vi "dataReferances.vi"(8 "error in (no error)":errorcluster) -> (0 "error out":errorcluster, 3 "?":T1)   [LabVIEW 2024]
uses:
  controls/dataRefs.ctl
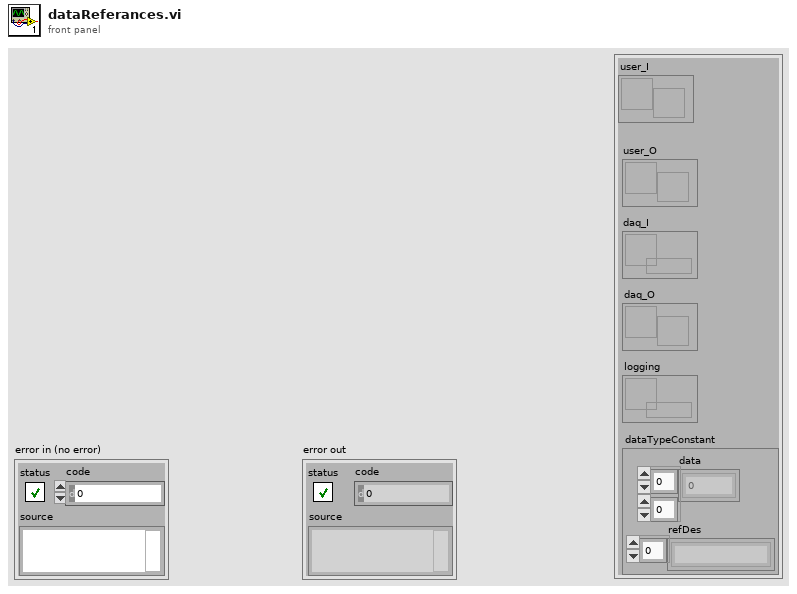
[diagram p1: front panel]
types:
  T1 = typedef "dataRefs.ctl" = cluster{"dataTypeConstant":cluster{"data":dbl[][], "refDes":string[]}, "user_I":refnum<notifier>, "user_O":refnum<notifier>, "daq_O":refnum<notifier>, "logging":refnum<queue>, "daq_I":refnum<queue>}
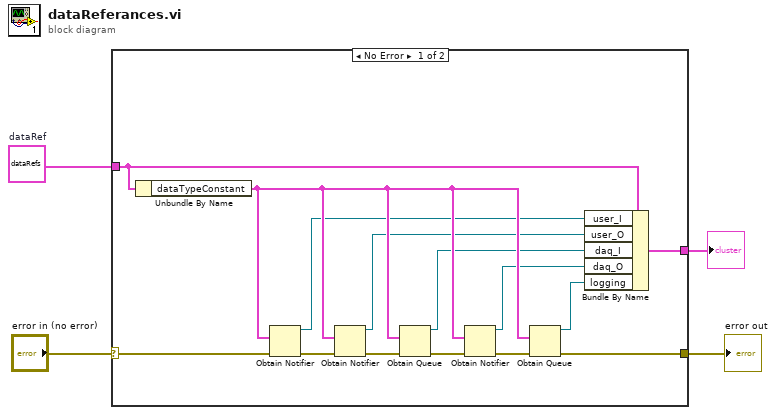
[diagram p0: block diagram]
diagram:
  w1 = T1 {"dataTypeConstant"={"data"=[], "refDes"=[]}, "user_I"=refnum, "user_O"=refnum, "daq_O"=refnum, "logging"=refnum, "daq_I"=refnum}  # dataRef
  n1 = case shown="No Error" "error in (no error)" {
    selector: "error in (no error)" -> [w18 w20]
    tunnel: [w17 w20] -> w3
    tunnel: [w12 w19] -> w2
    tunnel: w1 -> [w11 w19]
    frame No Error {
      n2 = Unbundle By Name(w11) -> ("dataTypeConstant"=w10:cluster{"data":dbl[][], "refDes":string[]})
      n3 = Obtain Notifier(notification data type=w10, error in (no error)=w18) -> (notifier out=w9:refnum<notifier>, error out=w16:errorcluster)  [unwired: 2 in, 1 out]
      n4 = Obtain Notifier(notification data type=w10, error in (no error)=w16) -> (notifier out=w8:refnum<notifier>, error out=w15:errorcluster)  [unwired: 2 in, 1 out]
      n5 = Obtain Queue(element data type=w10, error in (no error)=w15) -> (queue out=w6:refnum<queue>, error out=w14:errorcluster)  [unwired: 3 in, 1 out]
      n6 = Obtain Notifier(notification data type=w10, error in (no error)=w14) -> (notifier out=w7:refnum<notifier>, error out=w13:errorcluster)  [unwired: 2 in, 1 out]
      n7 = Obtain Queue(element data type=w10, error in (no error)=w13) -> (queue out=w5:refnum<queue>, error out=w17:errorcluster)  [unwired: 3 in, 1 out]
      n8 = Bundle By Name(cluster=w11, "user_I"=w9, "user_O"=w8, "daq_I"=w6, "daq_O"=w7, "logging"=w5) -> (w12:T1)
    }
    frame Error {
    }
  }
  "error out" <- w3
  "?" <- w2
